vi "Read B-Scan.vi"(8 "error in (no error)":errorcluster, 10 "Index":u32, 11 "Read in":refnum<class "Read.lvclass">) -> (0 "error out":errorcluster, 2 "Raw B-Scan":u16[][](array[numeric]), 3 "Read out":refnum<class "Read.lvclass">)   [LabVIEW 2014, in "Read.lvclass"]
uses:
  Read.lvclass
  Read.lvclass/Read.ctl
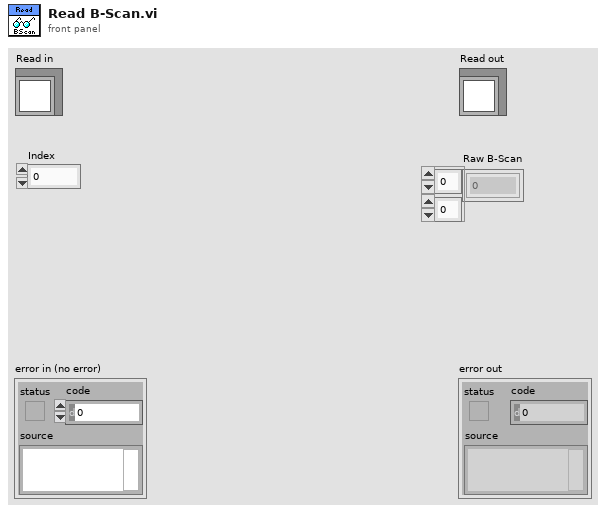
[diagram p1: front panel]
types:
  T1 = typedef "Read.lvclass/BScan.ctl" = cluster{"Points Per A-Scan":dbl, "A-Scans per B-Scan":dbl}
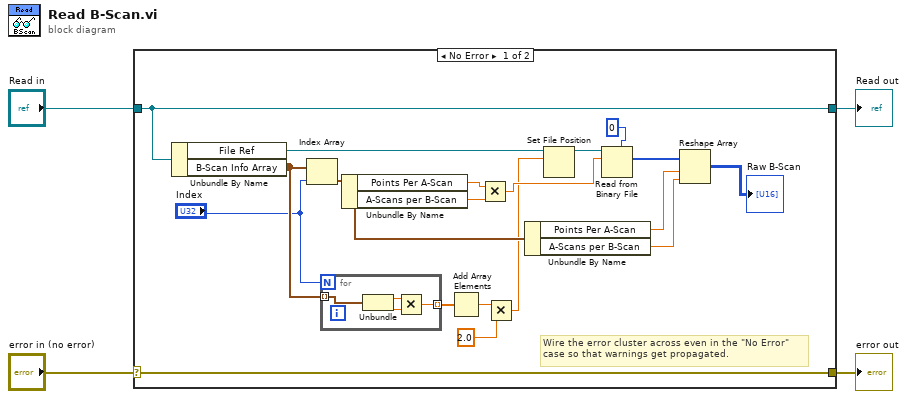
[diagram p0: block diagram]
diagram:
  n1 = case shown="No Error" "error in (no error)" {
    selector: "error in (no error)" -> [w23 w29]
    tunnel: [w23 w29] -> w3
    tunnel: [w22 w28] -> w1
    tunnel: "Read in" -> [w22 w28]
    frame No Error {
      # "Wire the error cluster across even in the \"No Error\"\ncase so that warnings get propagated."
      n2 = Unbundle By Name(w22) -> ("File Ref"=w20:refnum<file>, "B-Scan Info Array"=w10:T1[])
      n3 = Index Array(array=w10, index="Index") -> (element=w14:T1)
      n4 = for {
        N: "Index" -> [_]
        tunnel: w10 -> [w27] mode=indexing
        tunnel: [w24] -> w8 mode=indexing
        n5 = Unbundle(w27) -> ("Points Per A-Scan"=w26:dbl, "A-Scans per B-Scan"=w25:dbl)
        n6 = Multiply(x=w26, y=w25) -> (x*y=w24:dbl)
      }
      n7 = Unbundle By Name(w14) -> ("Points Per A-Scan"=w18:dbl, "A-Scans per B-Scan"=w19:dbl)
      n8 = Add Array Elements(numeric array=w8) -> (sum=w7:dbl)
      n9 = Multiply(x=w18, y=w19) -> (x*y=w17:dbl)
      n10 = Multiply(x=w7, y=2.0) -> (x*y=w5:dbl)
      n11 = Unbundle By Name(w14) -> ("Points Per A-Scan"=w13:dbl, "A-Scans per B-Scan"=w12:dbl)
      n12 = Set File Position(offset (in bytes) (0)=w5, refnum=w20) -> (refnum out=w21:refnum<file>)  [unwired: 2 in, 1 out]
      n13 = Read from Binary File(5:u16 0, 10:w17, 11:w21) -> (2:w15:u16[])  [unwired: 3 in, 3 out]
      n14 = Reshape Array(w15, w13, w12) -> (→"Raw B-Scan":u16[][])
    }
    frame Error {
    }
  }
  "error out" <- w3
  "Read out" <- w1
